vi "Read Digital Port.vi"(8 "error in (no error)":errorcluster, 11 "Digital IO Instrumentgital Input in":refnum<class "Digital IO Instrument.lvclass">) -> (0 "error out":errorcluster, 2 "DIs":bool[](array[boolean]), 3 "Digital IO Instrumentgital Input out":refnum<class "Digital IO Instrument.lvclass">)   [LabVIEW 2025, in "Digital IO.lvlib" / "Digital IO Instrument.lvclass"]
uses:
  Digital IO Instrument.lvclass
  Digital IO Instrument.lvclass/Digital IO Instrument.ctl
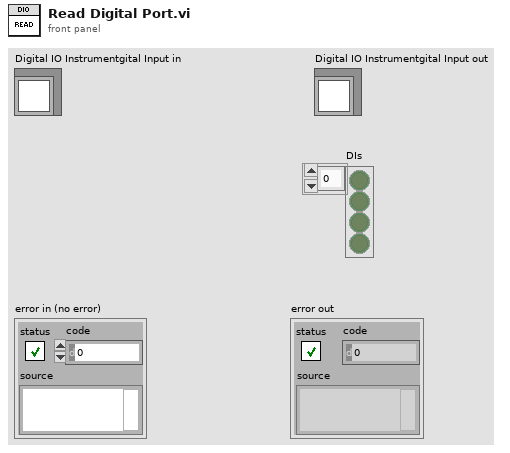
[diagram p1: front panel]
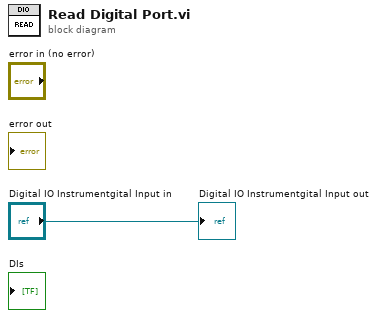
[diagram p0: block diagram]
diagram:
  "Digital IO Instrumentgital Input out" <- "Digital IO Instrumentgital Input in"
